vi "Fastlite5216_BuildError.vi"(8 "error in (no error)":errorcluster, 10 "Error source":string, 11 "Error Reason":u8(ring) format="x%02x" items=["unknown"=0, "invalid parameter"=1, "invalid password"=2, "invalid command"=3, "invalid size"=4, "meas pending"=5, "invalid pixel range"=6, "invalid int. time"=7, "operation not supported"=8, "invalid combination"=9, "no buffer available"=10, "no spectra available"=11, "invalid state"=12, "unexpected dma int"=13, "invalid fpga file"=14, "invalid firmware"=252, "spectrometer not found"=253, "timeout"=254, "unexpected response"=255]) -> (0 "error out":errorcluster)   [LabVIEW 2012, in "Fastlite5216-VIs.lvlib"]
doc: "This translates spectrometer internal error codes into LabVIEW error clusters. Generated error codes are in the 31000-31255 range."
uses:
  Fastlite5216-VIs.lvlib
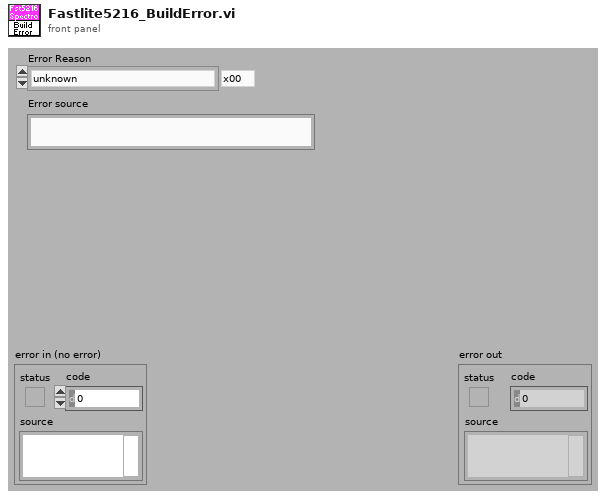
[diagram p1: front panel]
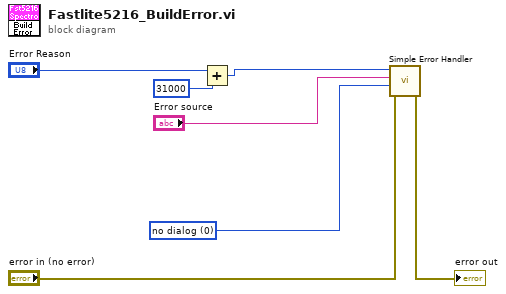
[diagram p0: block diagram]
diagram:
  w3 = u16 0 items=["no dialog", "OK message", "continue or stop message", "OK message + warnings", "continue/stop + warnings"] ("type of dialog (OK msg:1)")
  n1 = Add(x="Error Reason", y=31000) -> (x+y=w2:i32)
  n2 = call <vilib>:"Simple Error Handler.vi"("error code (no error:0)"=w2, "error source (\" \")"="Error source", "type of dialog (OK msg:1)"=w3, "error in (no error)"="error in (no error)") -> ("error out"=→"error out":errorcluster)  [unwired: 1 in, 4 out]
